vi "Set Columns.vi"(3 "error in (no error)":errorcluster, 4 "Columns in":refnum<class "Column.lvclass">[](array[class]), 5 "DDS in":refnum<class "DDS.lvclass">) -> (0 "error out":errorcluster, 1 "DDS out":refnum<class "DDS.lvclass">)   [LabVIEW 2013, in "DDS.lvclass"]
uses:
  DDS.lvclass
  ColumnVIs/Column/Column.lvclass
  <vilib>/Utility/error.llb/DialogType.ctl
  Device/Device.lvclass
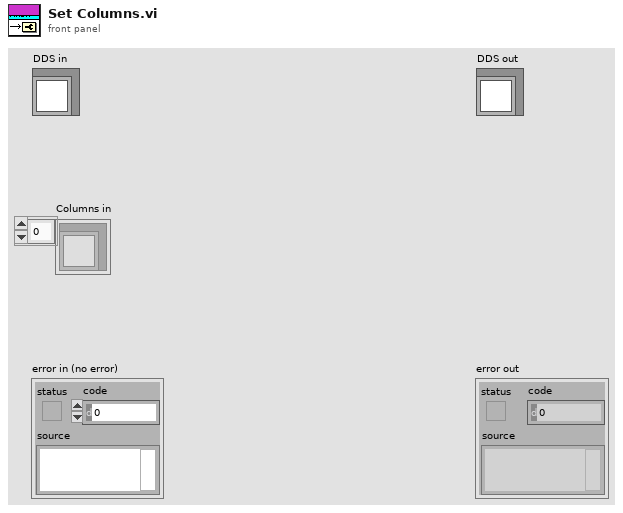
[diagram p1: front panel]
types:
  T1 = typedef "DialogType.ctl" = u16
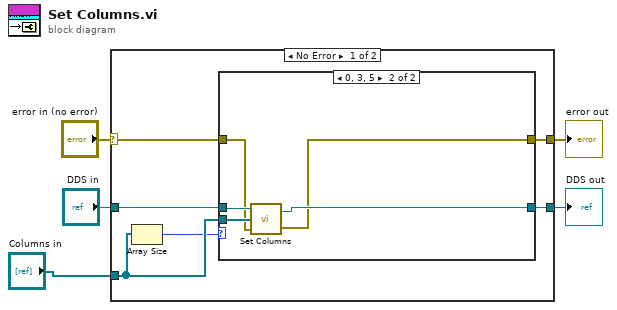
[diagram p0: block diagram]
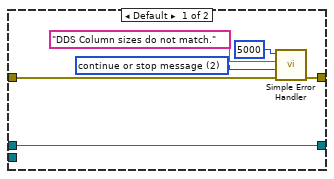
[diagram p2: hidden frame]
diagram:
  n1 = case shown="No Error" "error in (no error)" {
    selector: "error in (no error)" -> [w10 w23]
    tunnel: [w9 w23] -> w3
    tunnel: "DDS in" -> [w8 w24]
    tunnel: "Columns in" -> [w7 _]
    tunnel: [w11 w24] -> w2
    frame No Error {
      n2 = Array Size(array=w7) -> (size(s)=w6:i32)
      n3 = case shown="0, 3, 5" w6 {
        tunnel: w8 -> [w17 w22]
        tunnel: w7 -> [_ w21]
        tunnel: [w17 w20] -> w11
        tunnel: w10 -> [w16 w19]
        tunnel: [w15 w18] -> w9
        frame Default {
          w13 = T1 2 items=["no dialog", "OK message", "continue or stop message", "OK message + warnings", "continue/stop + warnings"] ("type of dialog (OK msg:1)")
          n4 = call <vilib>:"Simple Error Handler.vi"("error code (no error:0)"=5000, "error source (\" \")"="DDS Column sizes do not match." ("message"), "type of dialog (OK msg:1)"=w13, "error in (no error)"=w16) -> ("error out"=w15:errorcluster)  [unwired: 1 in, 4 out]
        }
        frame 0, 3, 5 {
          n5 = call-parent "Set Columns.vi"("error in (no error)"=w19, "Columns"=w21, "Device in"=w22) -> ("error out"=w18:errorcluster, "Device out"=w20:refnum<class "DDS.lvclass">)  [unwired: 1 in]
        }
      }
    }
    frame Error {
    }
  }
  "error out" <- w3
  "DDS out" <- w2
